vi "Publish If True.vi"(8 "error in (no error)":errorcluster, 9 "Data to Publish":bool, 10 "Datum Name":string, 11 "IModel in":refnum<class "IModel.lvclass">) -> (0 "error out":errorcluster, 3 "IModel out":refnum<class "IModel.lvclass">)   [LabVIEW 2020, in "IModel.lvlib" / "IModel.lvclass"]
doc: "仅当布尔值为TRUE时才发布该值。此发布允许多个参与者或多段代码发布一个标志，该标志在中介总线上保持为真，直到另一个参与者有意处理它。（全局标志设置的简单多对一选项）"
uses:
  IModel.lvclass
  IObserver/IObserver/IObserver.lvclass/IObserver.ctl
  IModel.lvclass/IModel.ctl
  IMediator/PublishRequest/PublishRequest.lvclass/PublishRequest.ctl
  IMediator/IMediator Messages/Publish Msg/Publish Msg.lvclass/Publish Msg.ctl
  composed-af-messages/Source/RoundTripMessage/RoundTripMessage.lvclass/RoundTripMessage.ctl
  <vilib>/ActorFramework/Message Enqueuer/Message Enqueuer.lvclass/Message Enqueuer.ctl
  IMediator/IMediator Messages/Publish Msg/Send Pre-Addressed Publish.vi
  IObserver/IObserver/Read Unique ID.vi
  IMediator/PublishRequest/Pack Publish Request.vi
  composed-af-messages/Source/RoundTripMessage/Return Round-Trip Message.vi
  <vilib>/ActorFramework/Message Enqueuer/Enqueue.vi
  IMediator/IMediator Messages/Publish Msg/Publish Msg.lvclass
  composed-af-messages/Source/RoundTripMessage/RoundTripMessage.lvclass
  C:/Program Files/National Instruments/LabVIEW 2020/vi.lib/ActorFramework/Message/Message.lvclass
  <vilib>/Utility/error.llb/Error Cluster From Error Code.vi
  <vilib>/ActorFramework/Message Priority Queue/Priority Enqueue.vi
  IMediator/PublishRequest/PublishRequest.lvclass
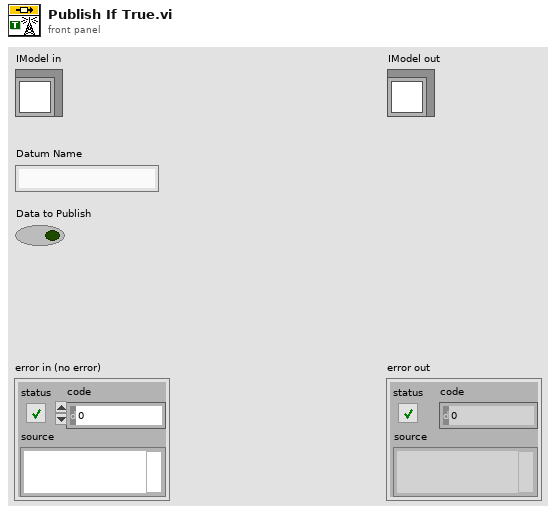
[diagram p1: front panel]
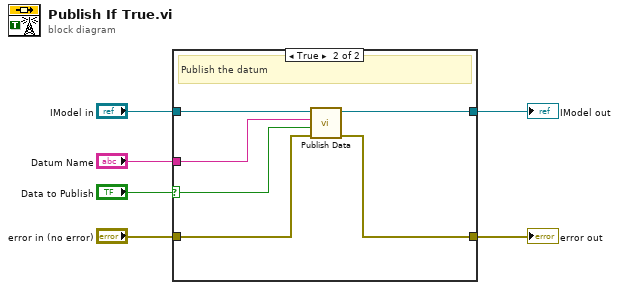
[diagram p0: block diagram]
diagram:
  n1 = case shown="True" "Data to Publish" {
    selector: "Data to Publish" -> [_ w9]
    tunnel: "IModel in" -> [w8 w14]
    tunnel: [w8 w13] -> w5
    tunnel: "error in (no error)" -> [w7 w12]
    tunnel: [w7 w11] -> w3
    tunnel: "Datum Name" -> [_ w10]
    frame False {
      # "...because it could clear prior state from the bus"
      # "Do not publish"
    }
    frame True {
      # "Publish the datum"
      n2 = call "Publish Data.vi"("error in (no error)"=w12, "Data to Publish"=w9, "Datum Name"=w10, "IModel in"=w14) -> ("error out"=w11:errorcluster, "IModel out"=w13:refnum<class "IModel.lvclass">)  [unwired: 6 in]
    }
  }
  "IModel out" <- w5
  "error out" <- w3
